vi "Calibration Unlock.vi"(8 "error in (no error)":errorcluster, 10 "Password":string, 11 "VISA resource name":refnum<visa-resource-name>="GPIB0::24::INSTR") -> (0 "error out":errorcluster, 3 "VISA resource name out":refnum<visa-resource-name>)   [LabVIEW 2015, in "Keithley 2450.lvlib"]
doc: "This VI unlocks calibration functions."
uses:
  <instrlib>/Keithley 2450/Keithley 2450.lvlib
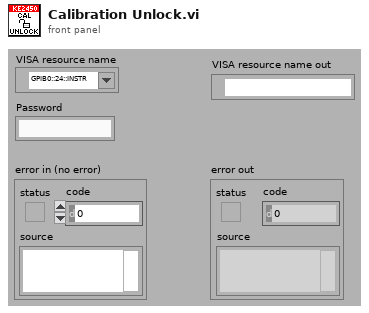
[diagram p1: front panel]
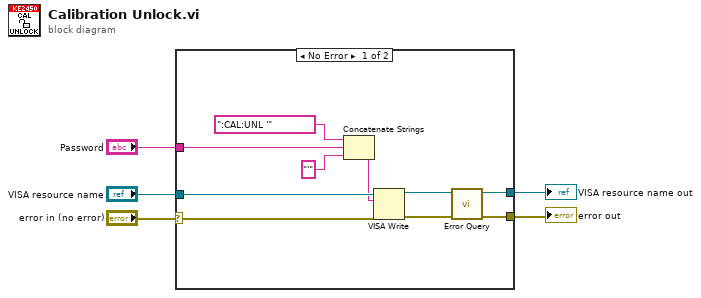
[diagram p0: block diagram]
diagram:
  n1 = case shown="No Error" "error in (no error)" {
    selector: "error in (no error)" -> [w15 w17]
    tunnel: [w9 w17] -> w4
    tunnel: "VISA resource name" -> [w14 w16]
    tunnel: "Password" -> [w13 _]
    tunnel: [w8 w16] -> w1
    frame No Error {
      n2 = Concatenate Strings(":CAL:UNL '" ("string"), w13, "'") -> (w11:string)
      n3 = VISA Write(VISA resource name=w14, write buffer=w11, error in (no error)=w15) -> (VISA resource name out=w7:refnum<visa-resource-name>, error out=w6:errorcluster)  [unwired: 1 out]
      n4 = call <instrlib>:"Error Query.vi"("error in (no error)"=w6, "VISA resource name"=w7) -> ("error out"=w9:errorcluster, "VISA resource name out"=w8:refnum<visa-resource-name>)  [unwired: 6 in, 2 out]
    }
    frame Error {
      # "Do nothing if error condition"
    }
  }
  "error out" <- w4
  "VISA resource name out" <- w1
